vi "3 Column Sort.vi"(6 "Tertiary Column":i32, 9 "Secondary Column":i32, 10 "Primary Column":i32, 11 "3 Column Array":dbl[][](array[numeric])) -> (3 "Sorted Array":dbl[][](array[numeric]))   [LabVIEW 2013]
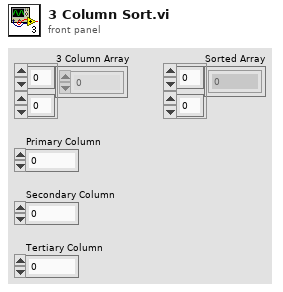
[diagram p1: front panel]
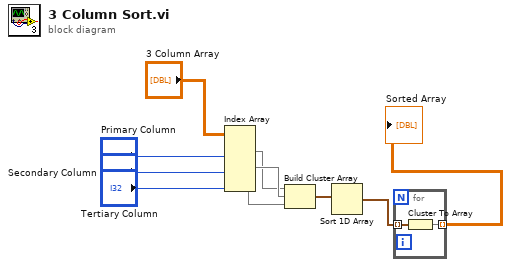
[diagram p0: block diagram]
diagram:
  n1 = Index Array(array="3 Column Array", index (col) #1="Primary Column", index (col) #2="Secondary Column", index (col) #3="Tertiary Column") -> (element #1=w5:dbl[], element #2=w6:dbl[], element #3=w7:dbl[])  [unwired: 3 in]
  n2 = Build Cluster Array(w5, w6, w7) -> (w8:cluster{dbl, dbl, dbl}[])
  n3 = Sort 1D Array(array=w8) -> (sorted array=w9:cluster{dbl, dbl, dbl}[])
  n4 = for {
    tunnel: w9 -> [w12] mode=indexing
    tunnel: [w11] -> w10 mode=indexing
    n5 = Cluster To Array(cluster=w12) -> (array=w11:dbl[])
  }
  "Sorted Array" <- w10
